vi "search_peak.vi"(4 "Max Channel":i32, 6 "Min Channel":i32, 9 "width":i32=3 min=3, 10 "threshold":dbl format="%0.2f", 11 "Spectrum":dbl[](array[numeric])) -> (1 "Best 8":i32[][](array[numeric]), 2 "peaks found":i32, 3 "set max":cluster{"Channels":dbl[], "Intensity":dbl[]})   [LabVIEW 2023]
uses:
  <vilib>/Analysis/1siggen.llb/Ramp Pattern by Samples.vi
  <vilib>/Analysis/NI_AALBase.lvlib
  <vilib>/Analysis/NI_AAL_SigProc.lvlib
panel:
  out "transposed array":i32[][](array[numeric])
  out "subarray":i64[][](array[numeric])
  out "Array":i64[][](array[numeric])
  out "XY Graph":cluster{"Locations":dbl[], "Amplitudes":dbl[]}[](graph)
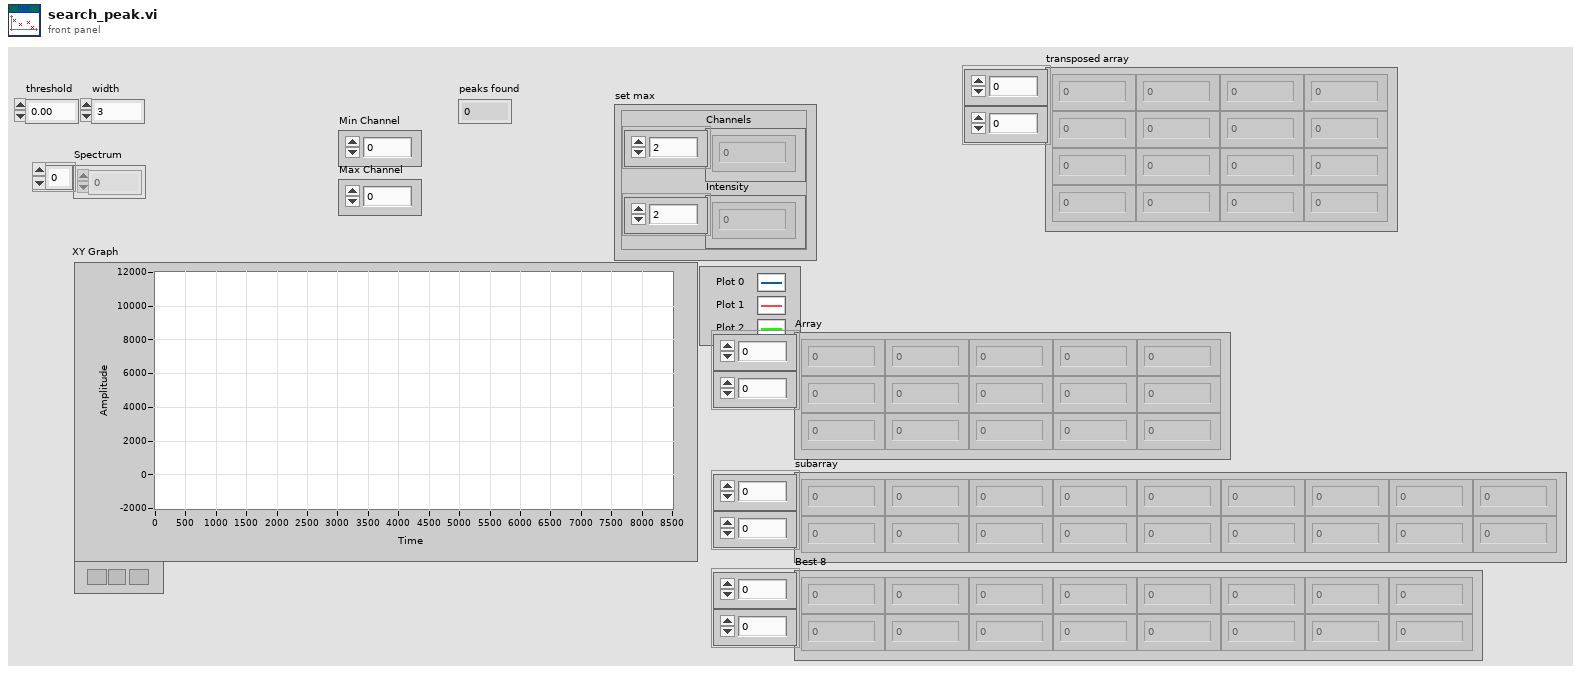
[diagram p1: front panel]
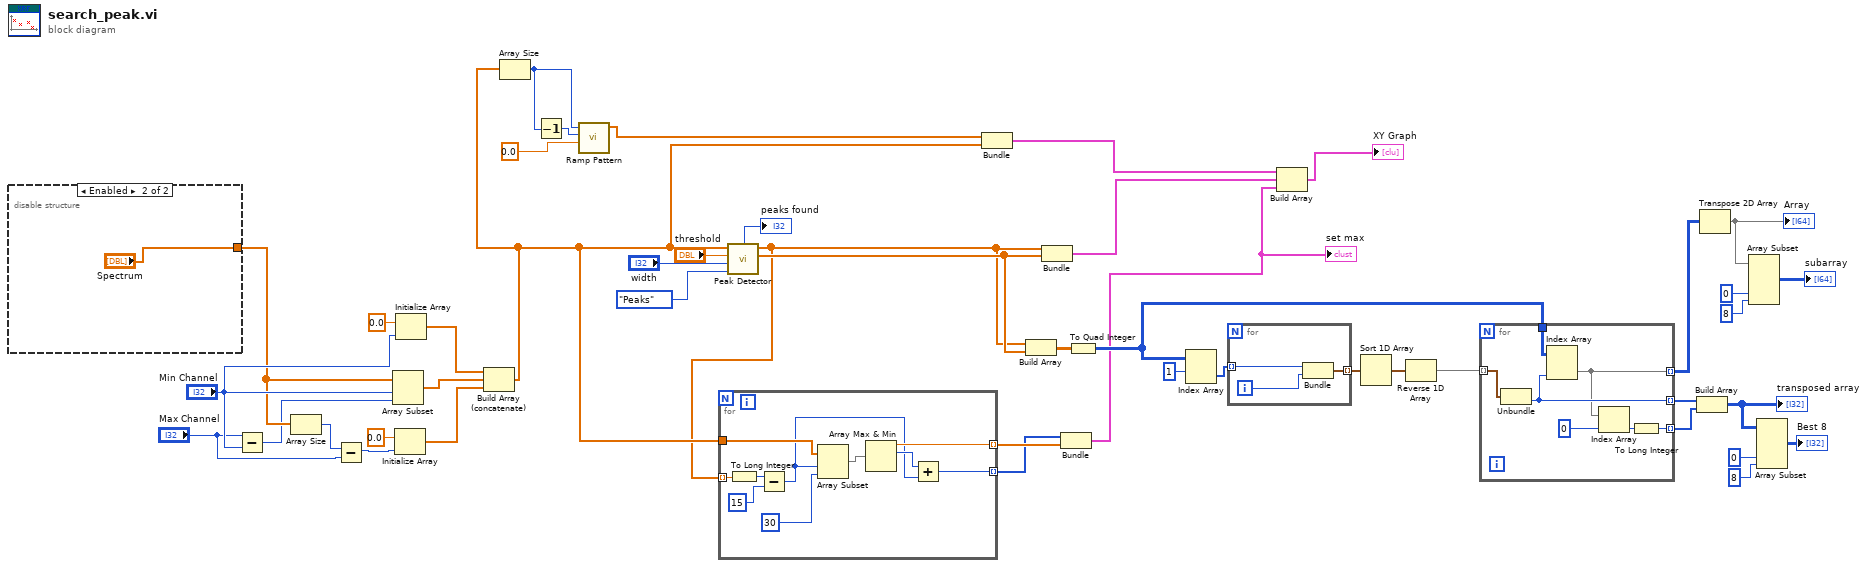
[diagram p0: block diagram]
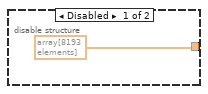
[diagram p2: hidden frame]
diagram:
  n1 = disable-structure shown="Enabled" {
    disable-tunnel: [dbl[] array[8193 elements] ("Spectrum 2") "Spectrum"] -> w33
    frame Disabled {
    }
    frame Enabled {
    }
  }
  n2 = Subtract(x="Max Channel", y="Min Channel") -> (x-y=w31:i32)
  n3 = Array Size(array=w33) -> (size(s)=w32:i32)
  n4 = Subtract(x=w32, y="Max Channel") -> (x-y=w29:i32)
  n5 = Array Subset(array=w33, index="Min Channel", length=w31) -> (w26:dbl[])
  n6 = Initialize Array(0.0 ("element"), w29) -> (w25:dbl[])
  n7 = Initialize Array(0.0 ("element"), "Min Channel") -> (w27:dbl[])
  n8 = Build Array (concatenate)(w27, w26, w25) -> (w5:dbl[])
  n9 = Array Size(array=w5) -> (size(s)=w37:i32)
  n10 = Decrement(x=w37) -> (x-1=w38:i32)
  n11 = call-poly <vilib>:"Ramp Pattern.vi"("start"=0.0, "end"=w38, "samples"=w37) -> ("Ramp Pattern"=w36:dbl[])  [unwired: 7 in, 1 out]
  n12 = call <vilib>:"Peak Detector.vi"("peaks/valleys"=enum32{"Peaks", "Valleys"}."Peaks", "width"="width", "threshold"="threshold", "X"=w5) -> ("Amplitudes"=w24:dbl[], "Locations"=w4:dbl[], "# found"=→"peaks found":i32)  [unwired: 3 in, 2 out]
  n13 = for {
    tunnel: w5 -> [w55]
    tunnel: w4 -> [w50] mode=indexing
    tunnel: [w53] -> w3 mode=indexing
    tunnel: [w51] -> w2 mode=indexing
    n14 = To Long Integer(number=w50) -> (32bit integer=w57:i32)
    n15 = Subtract(x=w57, y=15) -> (x-y=w49:i32)
    n16 = Array Subset(array=w55, index=w49, length=30) -> (w54:dbl[])
    n17 = Array Max & Min(array=w54) -> (max value=w53:dbl, max index (indices)=w52:i32)  [unwired: 2 out]
    n18 = Add(x=w52, y=w49) -> (x+y=w51:i32)
  }
  n19 = Bundle("Ramp Pattern"=w36, w5) -> (w42:cluster{"Ramp Pattern":dbl[], dbl[]})  [unwired: 1 in]
  n20 = Build Array(w4, w24) -> (w13:dbl[][])
  n21 = Bundle("Locations"=w4, "Amplitudes"=w24) -> (w41:cluster{"Locations":dbl[], "Amplitudes":dbl[]})  [unwired: 1 in]
  n22 = Bundle(w2, w3) -> (w1:cluster{i32[], dbl[]})  [unwired: 1 in]
  "set max" <- w1
  n23 = To Quad Integer(1:w13) -> (0:w12:i64[][])
  n24 = Index Array(array=w12, index (row)=1 ("index")) -> (element=w20:i64[])  [unwired: 1 in]
  n25 = for {
    tunnel: [w60] -> w23 mode=indexing
    tunnel: w20 -> [w59] mode=indexing
    i -> [w61]
    n26 = Bundle(w59, w61) -> (w60:cluster{i64, i32})  [unwired: 1 in]
  }
  n27 = Build Array(w42, w41, w1) -> (→"XY Graph":cluster{"Locations":dbl[], "Amplitudes":dbl[]}[])
  n28 = Sort 1D Array(array=w23) -> (sorted array=w22:cluster{i64, i32}[])
  n29 = Reverse 1D Array(array=w22) -> (reversed array=w21:cluster{i64, i32}[])
  n30 = for {
    tunnel: w21 -> [w68] mode=indexing
    tunnel: w12 -> [w67]
    tunnel: [w65] -> w18 mode=indexing
    tunnel: [w66] -> w11 mode=indexing
    tunnel: [w62] -> w10 mode=indexing
    n31 = Unbundle(w68) -> (w66:i32)  [unwired: 1 out]
    n32 = Index Array(array=w67, index (col)=w66) -> (element=w65:i64[])  [unwired: 1 in]
    n33 = Index Array(array=w65, index=0) -> (element=w63:i64)
    n34 = To Long Integer(number=w63) -> (32bit integer=w62:i32)
  }
  n35 = Build Array(w11, w10) -> (w7:i32[][])
  "transposed array" <- w7
  n36 = Transpose 2D Array(2D array=w18) -> (transposed array=w17:i64[][])
  "Array" <- w17
  n37 = Array Subset(array=w17, index (col)=0 ("index"), length (col)=8 ("length")) -> (→"subarray":i64[][])  [unwired: 2 in]
  n38 = Array Subset(array=w7, index (col)=0 ("index"), length (col)=8 ("length")) -> (→"Best 8":i32[][])  [unwired: 2 in]
